vi "QSvgWidget.vi"(8 "Error In":errorcluster, 10 "file":string, 11 "Post-Bundled Subclass":refnum<class "QSvgWidget.lvclass">) -> (0 "Error Out":errorcluster, 3 "New QSvgWidget":refnum<class "QSvgWidget.lvclass">)   [LabVIEW 2014, in "QSvgWidget.lvclass"]
doc: "LabVIEW-specific documentation is not yet available. See <b>https://doc.qt.io/qt-5/qsvgwidget.html#QSvgWidget</b>"
uses:
  QSvgWidget.lvclass
  LQ Core/LQCoreEngine/_Internal/LQIdentity Registry Action.ctl
  LQ Core/LQIdentity/LQIdentity.lvclass/LQIdentity.ctl
  LQ Core/LQCoreEngine/LQCoreEngine.lvclass
  LQ Core/LQ Core.lvlib
  LQ Core/LQIdentity/LQIdentity.lvclass
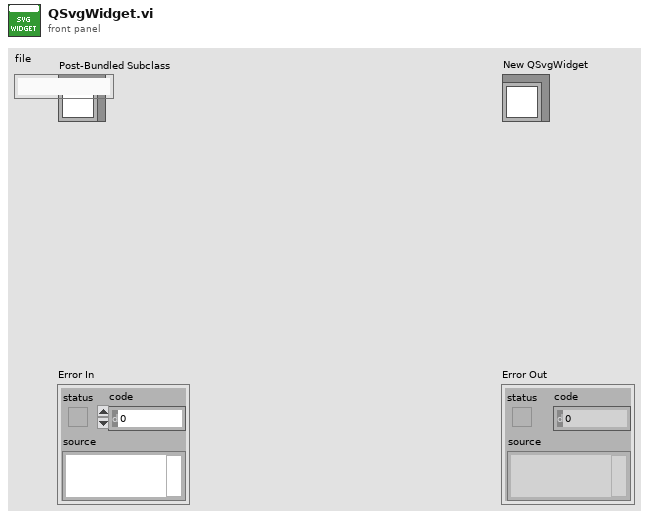
[diagram p1: front panel]
types:
  T1 = typedef "LQ Core.lvlib/LQCoreEngine.lvclass/LQIdentity Registry Action.ctl" = enum16{"Init", "Register LQIdentity", "Get LQIdentity Info", "Deregister LQIdentity"}
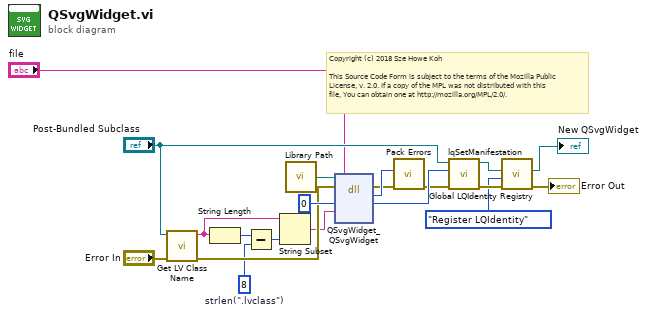
[diagram p0: block diagram]
diagram:
  w5 = 8  # strlen(".lvclass")
  # "Copyright (c) 2018 Sze Howe Koh\n\nThis Source Code Form is subject to the terms of the Mozilla Public\nLicense, v. 2.0. If a copy of the MPL was not distributed with this\nfile, You can obtain one at http://mozilla.org/MPL/2.0/."
  n1 = call <vilib>:"Get LV Class Name.vi"("error in (no error)"="Error In", "object"="Post-Bundled Subclass") -> ("error out"=w7:errorcluster, "class name"=w3:string)  [unwired: 8 in]
  n2 = String Length(string=w3) -> (length=w6:i32)
  n3 = Subtract(x=w6, y=w5) -> (x-y=w4:i32)
  n4 = String Subset(string=w3, length (rest)=w4) -> (substring=w2:string)  [unwired: 1 in]
  n5 = call "Library Path.vi"() -> ("Library Path"=w18:path)
  n6 = dll-call lib="?" fn="QSvgWidget_QSvgWidget"(path in=w18, error in=w7, "_retVal"=u64 0 ("_instance"), "_className"=w2, "file"="file") -> (error out=w16:errorcluster, w17:i32, "_retVal"=w19:u64)  [unwired: 3 in, 1 out]
  n7 = call "Pack Errors.vi"("Error In"=w16, "Error Code"=w17) -> ("Error Out"=w15:errorcluster)  [unwired: 9 in]
  n8 = call "lqSetManifestation.vi"("Error In"=w15, "Manifestation"=w19, "LQIdentity in"="Post-Bundled Subclass") -> ("Error Out"=w13:errorcluster, "LQIdentity out"=w14:refnum<class "QSvgWidget.lvclass">)  [unwired: 7 in]
  n9 = call "Global LQIdentity Registry.vi"("Error In"=w13, "Registry Action"=LQIdentity_Registry_Action."Register LQIdentity", "LQIdentity Info In"=w14) -> ("Error Out"=→"Error Out":errorcluster, "LQIdentity Info Out"=→"New QSvgWidget":refnum<class "QSvgWidget.lvclass">)  [unwired: 7 in]
